vi "Error Clear.vi"(4 "wait(ms)":u32, 6 "error in":errorcluster) -> (1 "error in (no error)":errorcluster)   [LabVIEW 2015]
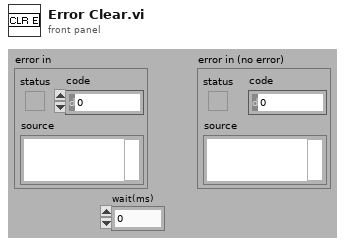
[diagram p1: front panel]
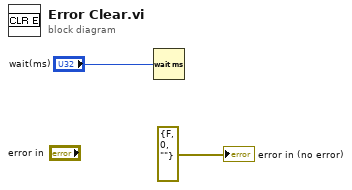
[diagram p0: block diagram]
diagram:
  n1 = Wait (ms)(milliseconds to wait="wait(ms)") -> ()  [unwired: 1 out]
  "error in (no error)" <- errorcluster {"status"=FALSE, "code"=0, "source"=""} ("error in (no error)")
